vi "PLC_OP10_Read.vi"(8 "error in (no error)":errorcluster, 11 "S7 Connection in":T1) -> (0 "error out":errorcluster, 3 "S7 Connection out":T1)   [LabVIEW 2017]
uses:
  <vilib>/DATA AHEAD/SP7/typedefs/S7 Connection.ctl
  <vilib>/DATA AHEAD/SP7/typedefs/PLC Type.ctl
  <vilib>/DATA AHEAD/SP7/functions/read/read Dint array.vi
  <vilib>/DATA AHEAD/SP7/functions/read/read real array.vi
  <vilib>/DATA AHEAD/SP7/functions/read/read String.vi
  <vilib>/DATA AHEAD/SP7/SP7.lvlib
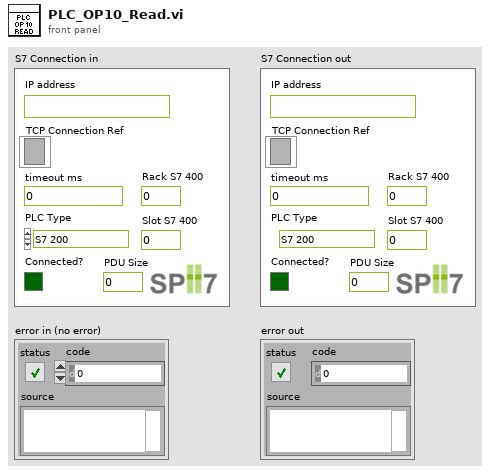
[diagram p1: front panel]
types:
  T1 = typedef "SP7.lvlib/S7 Connection.ctl" = cluster{"TCP Connection Ref":refnum<k5>, "IP address":string, "timeout ms":i32, "Connected?":bool, "PLC Type":T2, "Rack S7 400":u8, "Slot S7 400":u8, "PDU Size":u16, "connection semaphore":T3}
  T2 = typedef "SP7.lvlib/PLC Type.ctl" = enum16{"S7 200", "S7 300/400", "S7 1200", "S7 1500", "LOGO!8"}
  T3 = typedef "Semaphore RefNum" = refnum<k1>
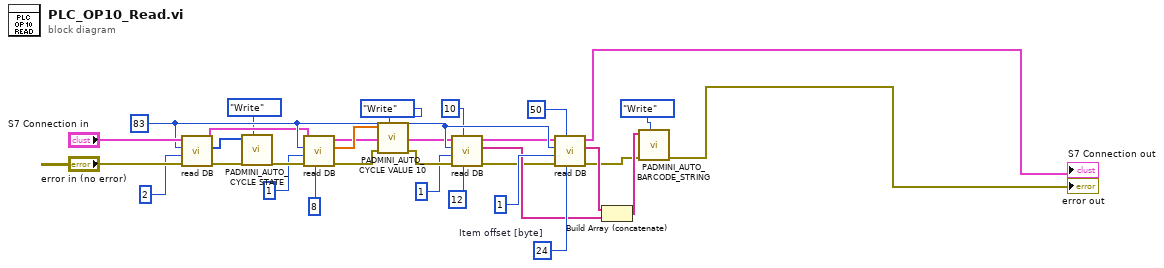
[diagram p0: block diagram]
diagram:
  w27 = u32 24  # Item offset [byte]
  w25 = u16 83 ("Data Block #")
  n1 = call-poly <vilib>:"read DB.vi"("error in (no error)"="error in (no error)", "items #"=u16 2 ("Items # [byte]"), "Data Block #"=w25, "S7 Connection in"="S7 Connection in") -> ("error out"=w2:errorcluster, "DINT result array"=w4:i32[], "S7 Connection out"=w7:T1)  [unwired: 5 in]
  n2 = call "PADMINI_AUTO_CYCLE STATE.vi"("Enum"=enum16{"Read", "Write"}."Write", "error in (no error)"=w2, "Input"=w4) -> ("error out"=w6:errorcluster)  [unwired: 7 in, 1 out]
  n3 = call-poly <vilib>:"read DB.vi"("Item offset [byte]"=u32 8, "error in (no error)"=w6, "items #"=u16 1 ("Items # [byte]"), "Data Block #"=w25, "S7 Connection in"=w7) -> ("error out"=w14:errorcluster, "REAL result array"=w16:sgl[], "S7 Connection out"=w8:T1)  [unwired: 4 in]
  n4 = call "PADMINI_AUTO_CYCLE VALUE 10.vi"("Enum"=enum16{"Read", "Write"}."Write", "error in (no error)"=w14, "Input"=w16) -> ("error out"=w15:errorcluster)  [unwired: 7 in, 1 out]
  n5 = call-poly <vilib>:"read DB.vi"("Item offset [byte]"=u32 12, "String length reserved in DB (default=254)"=u16 10, "error in (no error)"=w15, "items #"=u16 1 ("Items # [byte]"), "Data Block #"=w25, "S7 Connection in"=w8) -> ("error out"=w18:errorcluster, "STRING result Array"=w21:string[], "S7 Connection out"=w17:T1)  [unwired: 2 in, 1 out]
  n6 = call-poly <vilib>:"read DB.vi"("Item offset [byte]"=w27, "String length reserved in DB (default=254)"=u16 50, "error in (no error)"=w18, "items #"=u16 1 ("Items # [byte]"), "Data Block #"=w25, "S7 Connection in"=w17) -> ("error out"=w19:errorcluster, "STRING result Array"=w23:string[], "S7 Connection out"=→"S7 Connection out":T1)  [unwired: 2 in, 1 out]
  n7 = Build Array (concatenate)(w23, w21) -> (w22:string[])
  n8 = call "PADMINI_AUTO_BARCODE_STRING.vi"("Enum"=enum16{"Read", "Write"}."Write", "error in (no error)"=w19, "Input"=w22) -> ("error out"=→"error out":errorcluster)  [unwired: 7 in, 1 out]
